vi "Send Error.vi"(7 "Interactive?":bool=TRUE, 8 "error in (no error)":errorcluster) -> (0 "error out":errorcluster, 2 "Stop?":bool)   [LabVIEW 2015, in "Mag Lab Error Handler.lvlib" / "Mag Lab Error Handler.lvclass"]
uses:
  Mag Lab Error Handler.lvclass
  Mag Lab Error Handler Messages/Handle System Error Msg/Handle System Error Msg.lvclass/Handle System Error Msg.ctl
  <vilib>/ActorFramework/Message Enqueuer/Message Enqueuer.lvclass/Message Enqueuer.ctl
  <vilib>/ActorFramework/Message Enqueuer/Enqueue.vi
  <vilib>/ActorFramework/Message Priority Queue/Priority Enqueue.vi
  Mag Lab Error Handler Messages/Handle System Error Msg/Handle System Error Msg.lvclass
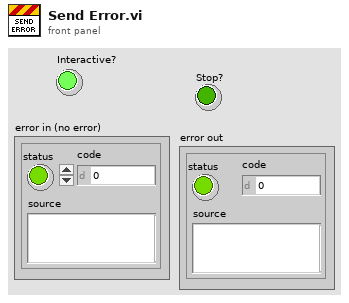
[diagram p1: front panel]
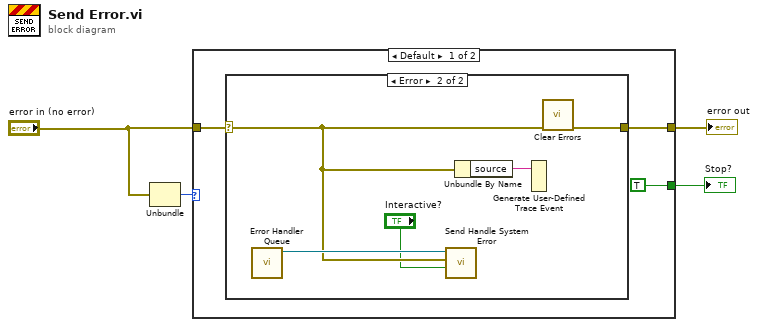
[diagram p0: block diagram]
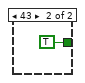
[diagram p3: hidden frame]
diagram:
  n1 = Unbundle("error in (no error)") -> ("code"=w2:i32)  [unwired: 2 out]
  n2 = case shown="Default" w2 {
    tunnel: [TRUE ("Stop?") TRUE ("Stop?")] -> w4
    tunnel: "error in (no error)" -> [w5 _]
    tunnel: [w6 _] -> w1
    frame Default {
      n3 = case shown="Error" w5 {
        selector: w5 -> [w8 w10]
        tunnel: [w8 w12] -> w6
        frame No Error {
        }
        frame Error {
          n4 = call "Error Handler Queue.vi"() -> ("Error Handler Queue Out"=w11:refnum<class "Message Enqueuer.lvclass">)  [unwired: 11 in]
          n5 = call "Send Handle System Error.vi"("Interactive?"="Interactive?", "error to handle"=w10, "Message Enqueuer"=w11) -> ()  [unwired: 7 in, 2 out]
          n6 = Unbundle By Name(w10) -> ("source"=w13:string)
          n7 = Generate User-Defined Trace Event(2:w13) -> ()  [unwired: 1 in]
          n8 = call <vilib>:"Clear Errors.vi"("error in (no error)"=w10) -> ("error out"=w12:errorcluster)  [unwired: 5 in, 1 out]
        }
      }
    }
    frame 43 {
    }
  }
  "error out" <- w1
  "Stop?" <- w4
